vi "Open Existing TDMS File.vi"(8 "Error In":errorcluster, 11 "TDMS File Path":path) -> (0 "Error Out":errorcluster, 3 "TDMS File Ref Out":refnum<k34>)   [LabVIEW 2014]
doc: "Open an existing TDMS File."
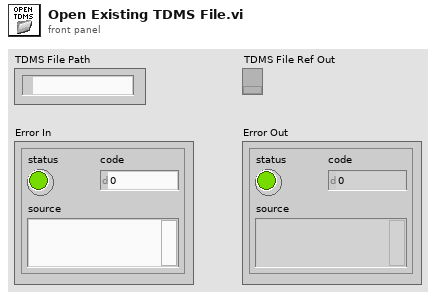
[diagram p1: front panel]
types:
  T1 = enum16{"open", "open or create", "create or replace", "create", "open (read-only)"}
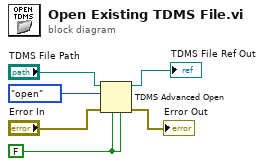
[diagram p0: block diagram]
diagram:
  w1 = FALSE ("enable asynchronous? (T)")
  n1 = TDMS Advanced Open(4:w1, 6:w1, 8:"Error In", 10:T1."open" ("operation (0:open)"), 11:"TDMS File Path") -> (0:→"Error Out":errorcluster, 3:→"TDMS File Ref Out":refnum<k34>)  [unwired: 1 out]
